vi "New Items.vi"(8 "error in (no error)":errorcluster, 10 "New Items":refnum<class "BetterItem.lvclass">[](array[class]), 11 "BetterBoxHandle in":refnum<class "BetterBoxHandle.lvclass">) -> (0 "error out":errorcluster, 3 "BetterBoxHandle out":refnum<class "BetterBoxHandle.lvclass">)   [LabVIEW 2020, in "BetterDragAndDrop.lvlib" / "BetterBoxHandle.lvclass"]
uses:
  BetterBoxHandle.lvclass
  C:/DSCE code/Open-source/betterdraganddrop_GIT/Source/Classes/BetterHandle/BetterHandle.lvclass
  BetterTreeItem/BetterItem.lvclass
  BetterTreeItem/BetterItem.lvclass/BetterItem.ctl
  BetterHandle/BetterHandle.lvclass/BetterHandle.ctl
  BetterHandle/BetterHandle.lvclass
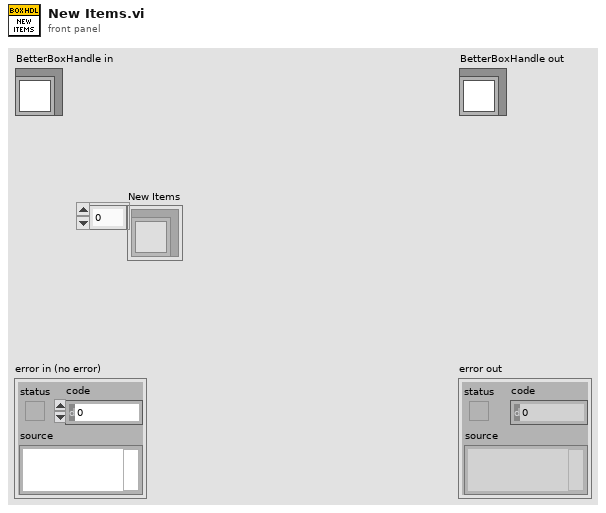
[diagram p1: front panel]
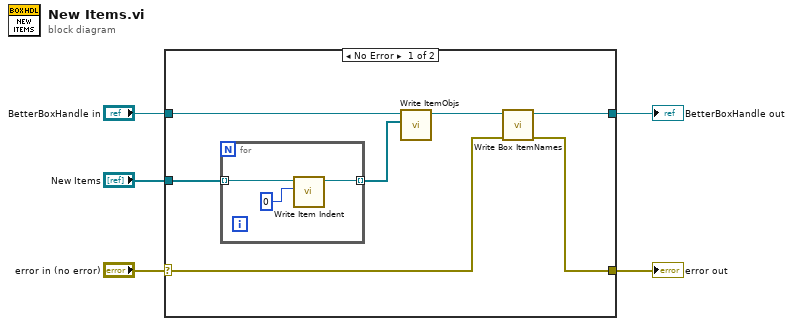
[diagram p0: block diagram]
diagram:
  n1 = case shown="No Error" "error in (no error)" {
    selector: "error in (no error)" -> [w10 w17]
    tunnel: [w9 w17] -> w4
    tunnel: "BetterBoxHandle in" -> [w7 w16]
    tunnel: [w8 w16] -> w5
    tunnel: "New Items" -> [w12 _]
    frame No Error {
      n2 = for {
        tunnel: [w13] -> w6 mode=indexing
        tunnel: w12 -> [w15] mode=indexing
        n3 = call "Write Item Indent.vi"("Item Indent"=0, "BetterTreeItem in"=w15) -> ("BetterTreeItem out"=w13:refnum<class "BetterItem.lvclass">)  [unwired: 9 in]
      }
      n4 = call "Write ItemObjs.vi"("ItemObjs"=w6, "BetterHandle in"=w7) -> ("BetterHandle out"=w11:refnum<class "BetterBoxHandle.lvclass">)  [unwired: 9 in]
      n5 = call-dynamic "Write Box ItemNames.vi"("error in (no error)"=w10, "BetterBoxHandle in"=w11) -> ("error out"=w9:errorcluster, "BetterBoxHandle out"=w8:refnum<class "BetterBoxHandle.lvclass">)  [unwired: 8 in]
    }
    frame Error {
    }
  }
  "error out" <- w4
  "BetterBoxHandle out" <- w5
